vi "adjust_motor_positions.vi"(0 "VISA Refnum in":refnum<visa-resource-name>, 4 "z position":dbl, 5 "y position":dbl, 6 "x position":dbl, 7 "r position":dbl, 8 "set z position":dbl, 9 "set y position":dbl, 10 "set x position":dbl, 11 "set r position":dbl) -> (3 "VISA Handle out":refnum<visa-resource-name>)   [LabVIEW 2025]
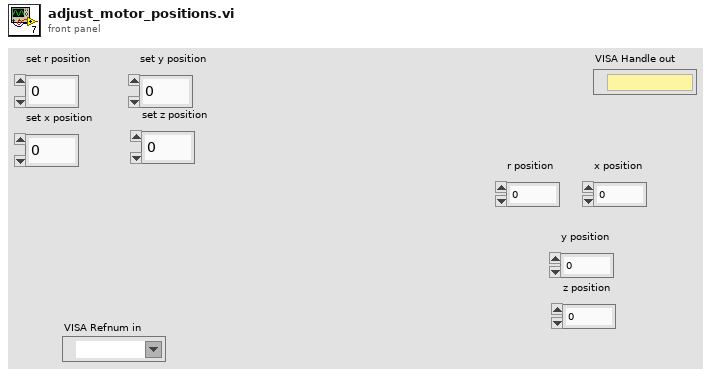
[diagram p1: front panel]
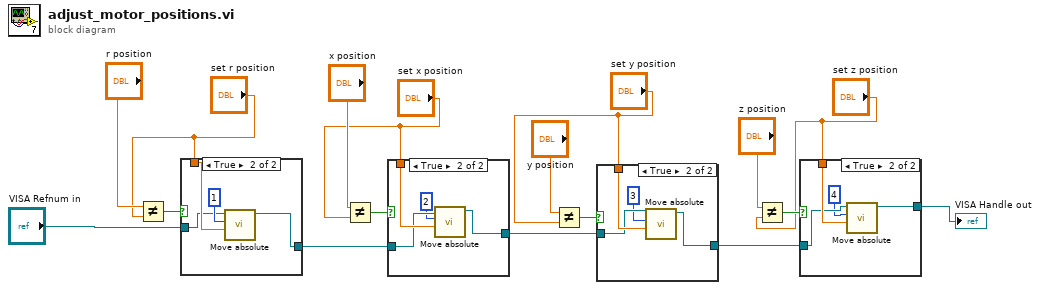
[diagram p0: block diagram]
diagram:
  n1 = Not Equal?(x="r position", y="set r position") -> (x != y?=w17:bool)
  n2 = case shown="True" w17 {
    tunnel: "set r position" -> [_ w22]
    tunnel: "VISA Refnum in" -> [w18 w20]
    tunnel: [w18 w19] -> w4
    frame False {
    }
    frame True {
      n3 = call <userlib>:"Move absolute.vi"("New target position (units)"=w22, "Axis in"=1, "VISA Handle in"=w20) -> ("VISA Handle out"=w19:refnum<visa-resource-name>)  [unwired: 3 in, 3 out]
    }
  }
  n4 = Not Equal?(x="x position", y="set x position") -> (x != y?=w16:bool)
  n5 = case shown="True" w16 {
    tunnel: "set x position" -> [_ w27]
    tunnel: w4 -> [w23 w26]
    tunnel: [w23 w25] -> w3
    frame False {
    }
    frame True {
      n6 = call <userlib>:"Move absolute.vi"("New target position (units)"=w27, "Axis in"=2, "VISA Handle in"=w26) -> ("VISA Handle out"=w25:refnum<visa-resource-name>)  [unwired: 3 in, 3 out]
    }
  }
  n7 = Not Equal?(x="y position", y="set y position") -> (x != y?=w15:bool)
  n8 = case shown="True" w15 {
    tunnel: "set y position" -> [_ w32]
    tunnel: w3 -> [w28 w31]
    tunnel: [w28 w30] -> w2
    frame False {
    }
    frame True {
      n9 = call <userlib>:"Move absolute.vi"("New target position (units)"=w32, "Axis in"=3, "VISA Handle in"=w31) -> ("VISA Handle out"=w30:refnum<visa-resource-name>)  [unwired: 3 in, 3 out]
    }
  }
  n10 = Not Equal?(x="z position", y="set z position") -> (x != y?=w14:bool)
  n11 = case shown="True" w14 {
    tunnel: "set z position" -> [_ w37]
    tunnel: w2 -> [w33 w36]
    tunnel: [w33 w35] -> w1
    frame False {
    }
    frame True {
      n12 = call <userlib>:"Move absolute.vi"("New target position (units)"=w37, "Axis in"=4, "VISA Handle in"=w36) -> ("VISA Handle out"=w35:refnum<visa-resource-name>)  [unwired: 3 in, 3 out]
    }
  }
  "VISA Handle out" <- w1
